vi "API.vi"() -> ()   [LabVIEW 2010]
uses:
  <vilib>/httpClient/LabVIEWHTTPClient.lvlib
panel:
  out "Temperature":string
  in  "CITY Box":string(combo)
  out "headers":string
  out "body":string
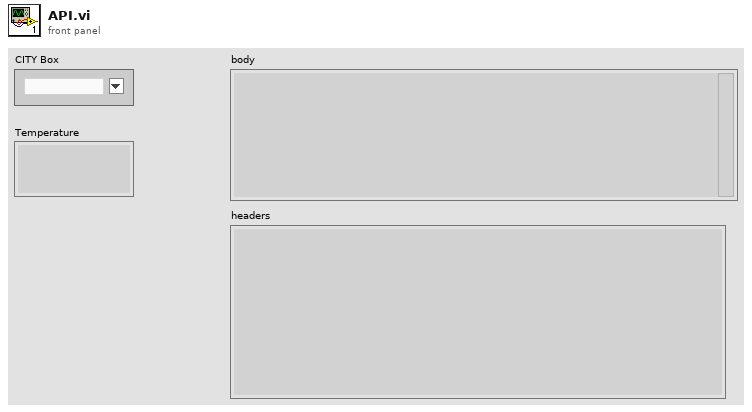
[diagram p1: front panel]
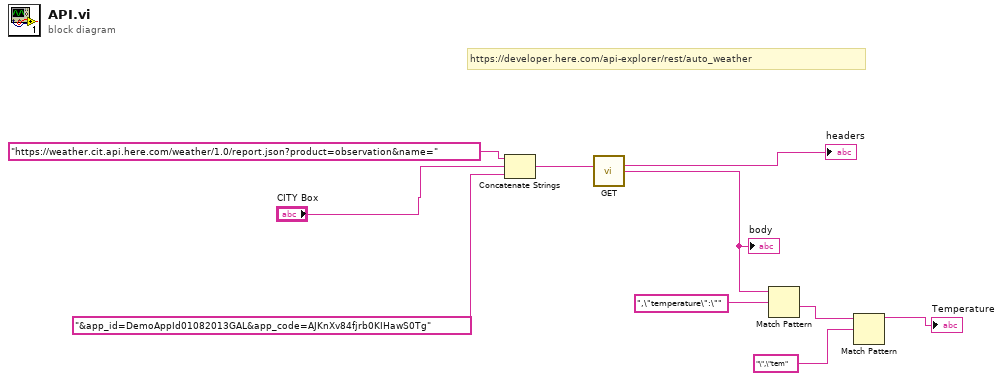
[diagram p0: block diagram]
diagram:
  # "https://developer.here.com/api-explorer/rest/auto_weather"
  n1 = Concatenate Strings("https://weather.cit.api.here.com/weather/1.0/report.json?product=observation&name=", "CITY Box", "&app_id=DemoAppId01082013GAL&app_code=AJKnXv84fjrb0KIHawS0Tg" ("string")) -> (w6:string)
  n2 = call <vilib>:"GET.vi"("url"=w6) -> ("headers"=→"headers":string, "body"=w5:string)  [unwired: 11 in, 2 out]
  "body" <- w5
  n3 = Match Pattern(string=w5, regular expression=",\"temperature\":\"") -> (after substring=w3:string)  [unwired: 1 in, 3 out]
  n4 = Match Pattern(string=w3, regular expression="\",\"tem") -> (before substring=→"Temperature":string)  [unwired: 1 in, 3 out]
